vi "9-2.vi"() -> ()   [LabVIEW 2019, in "9.lvlib"]
uses:
  9.lvlib
panel:
  out "sum":i32
  out "number":i32[][](array[numeric])
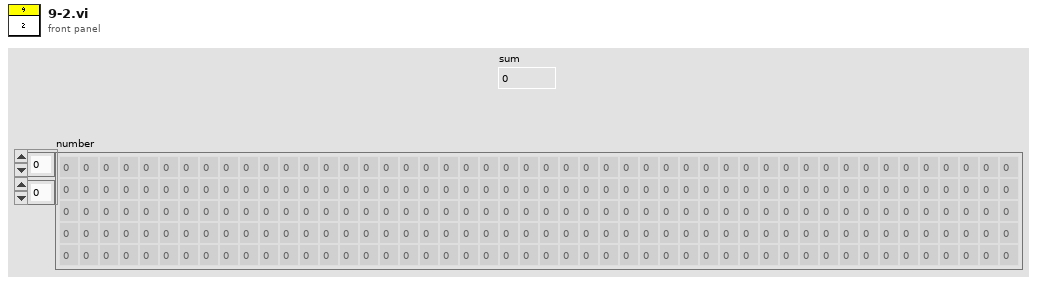
[diagram p1: front panel]
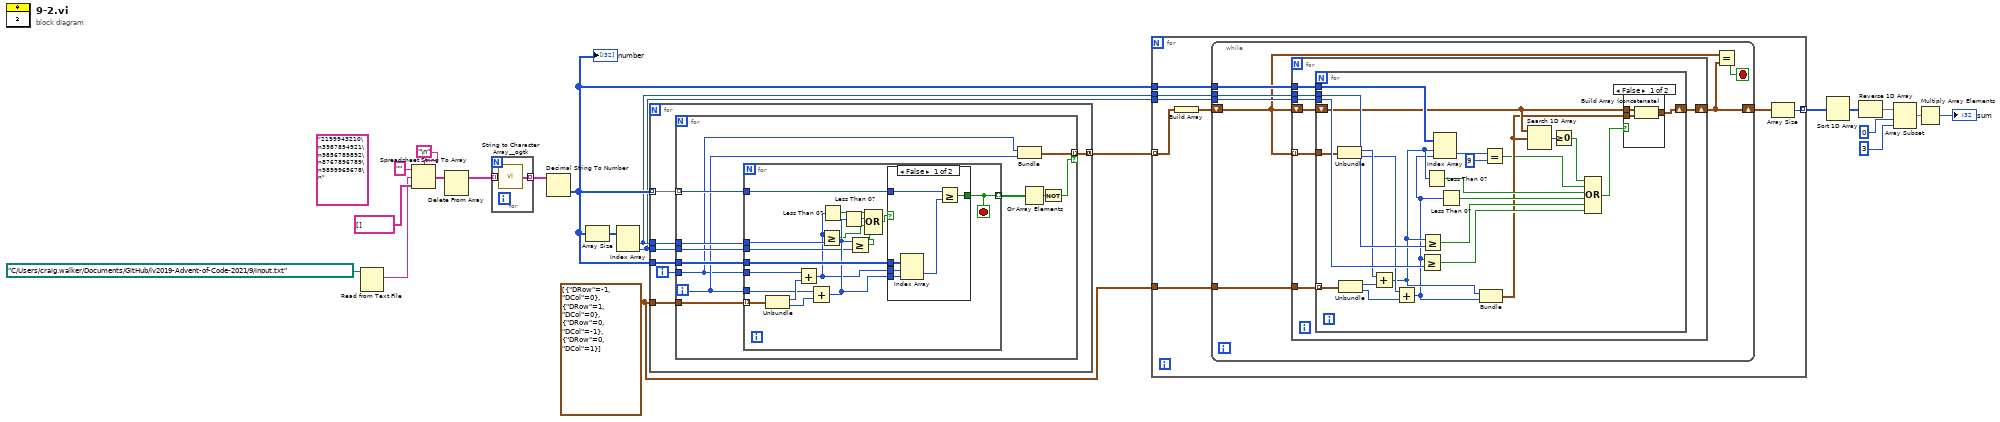
[diagram p0: block diagram]
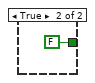
[diagram p3: hidden frame]
diagram:
  w9 = cluster{"DRow":i32, "DCol":i32}[] [{"DRow"=-1, "DCol"=0}, {"DRow"=1, "DCol"=0}, {"DRow"=0, "DCol"=-1}, {"DRow"=0, "DCol"=1}]
  (unwired) "2199943210\n3987894921\n9856789892\n8767896789\n9899965678\n"
  n1 = Read from Text File(file (use dialog)=path "C:/Users/craig.walker/Documents/GitHub/lv2019-Advent-of-Code-2021/9/input.txt") -> (text=w13:string)  [unwired: 3 in, 3 out]
  n2 = Spreadsheet String To Array(delimiter (Tab)="\n", format string="", spreadsheet string=w13, array type (2D Dbl)=string[] []) -> (array=w20:string[])
  n3 = Delete From Array(array=w20) -> (array with subset deleted=w14:string[])  [unwired: 2 in, 1 out]
  n4 = for {
    tunnel: w14 -> [w23] mode=indexing
    tunnel: [w22] -> w19 mode=indexing
    n5 = call <userlib>:"String to Character Array__ogtk.vi"("Input String"=w23) -> ("Character Array"=w22:string[])
  }
  n6 = Decimal String To Number(string=w19) -> (number=w12:i32[][])  [unwired: 2 in, 1 out]
  "number" <- w12
  n7 = Array Size(array=w12) -> (size(s)=w17:i32[])
  n8 = Index Array(array=w17) -> (element #1=w11:i32, element #2=w10:i32)  [unwired: 2 in]
  n9 = for {
    tunnel: w12 -> [w29] mode=indexing
    tunnel: w12 -> [w30]
    tunnel: w11 -> [w27]
    tunnel: w10 -> [w26]
    tunnel: w9 -> [w25]
    tunnel: [w24] -> w8 mode=concatenating
    i -> [w28]
    n10 = for {
      tunnel: w30 -> [w41]
      tunnel: w29 -> [w38] mode=indexing
      tunnel: w28 -> [w31]
      tunnel: w27 -> [w35]
      tunnel: w26 -> [w36]
      tunnel: w25 -> [w40]
      tunnel: [w32] -> w24 mode=indexing if=w34
      i -> [w33]
      n11 = for {
        tunnel: w41 -> [w50]
        tunnel: w31 -> [w56]
        tunnel: w33 -> [w54]
        tunnel: w40 -> [w58] mode=indexing
        tunnel: w38 -> [w48]
        tunnel: [w49] -> w39 mode=indexing
        tunnel: w36 -> [w46]
        tunnel: w35 -> [w45]
        stop <- w49 stop-if-true
        n12 = Unbundle(w58) -> ("DRow"=w57:i32, "DCol"=w55:i32)
        n13 = Add(x=w56, y=w57) -> (x+y=w44:i32)
        n14 = Add(x=w54, y=w55) -> (x+y=w47:i32)
        n15 = Greater Or Equal?(x=w44, y=w45) -> (x >= y?=w43:bool)
        n16 = Less Than 0?(x=w44) -> (x < 0?=w52:bool)
        n17 = Less Than 0?(x=w47) -> (x < 0?=w53:bool)
        n18 = Greater Or Equal?(x=w47, y=w46) -> (x >= y?=w42:bool)
        n19 = Compound Arithmetic op=OR(w52, w53, w43, w42) -> (w51:bool)
        n20 = case shown="False" w51 {
          tunnel: w48 -> [w64 _]
          tunnel: w50 -> [w63 _]
          tunnel: w44 -> [w62 _]
          tunnel: w47 -> [w61 _]
          tunnel: [w59 FALSE] -> w49
          frame False {
            n21 = Index Array(array=w63, index (row)=w62, index (col)=w61) -> (element=w60:i32)
            n22 = Greater Or Equal?(x=w64, y=w60) -> (x >= y?=w59:bool)
          }
          frame True {
          }
        }
      }
      n23 = Bundle(w31, w33) -> (w32:cluster{i32, i32})  [unwired: 1 in]
      n24 = Or Array Elements(Boolean array=w39) -> (logical OR=w37:bool)
      n25 = Not(x=w37) -> (.not. x?=w34:bool)
    }
  }
  n26 = for {
    tunnel: w8 -> [w69] mode=indexing
    tunnel: w12 -> [w73]
    tunnel: w11 -> [w72]
    tunnel: w10 -> [w71]
    tunnel: w9 -> [w70]
    tunnel: [w67] -> w7 mode=indexing
    n27 = Build Array(w69) -> (w68:cluster{i32, i32}[])
    n28 = while {
      tunnel: w73 -> [w80]
      tunnel: w72 -> [w79]
      tunnel: w71 -> [w78]
      tunnel: w70 -> [w77]
      shift-right: [w75] -> w66
      shift-left: w68 -> [w76]
      stop <- w74 stop-if-true
      n29 = for {
        tunnel: w80 -> [w87]
        tunnel: w79 -> [w86]
        tunnel: w78 -> [w85]
        tunnel: w77 -> [w84]
        tunnel: w76 -> [w81] mode=indexing
        shift-right: [w82] -> w75
        shift-left: w76 -> [w83]
        n30 = for {
          tunnel: w81 -> [w95]
          tunnel: w87 -> [w111]
          tunnel: w86 -> [w108]
          tunnel: w85 -> [w107]
          tunnel: w84 -> [w102] mode=indexing
          shift-right: [w97] -> w82
          shift-left: w83 -> [w96]
          n31 = Unbundle(w95) -> (w100:i32, w98:i32)
          n32 = Unbundle(w102) -> ("DRow"=w101:i32, "DCol"=w99:i32)
          n33 = Add(x=w100, y=w101) -> (x+y=w94:i32)
          n34 = Add(x=w98, y=w99) -> (x+y=w93:i32)
          n35 = Greater Or Equal?(x=w93, y=w107) -> (x >= y?=w103:bool)
          n36 = Greater Or Equal?(x=w94, y=w108) -> (x >= y?=w105:bool)
          n37 = Less Than 0?(x=w94) -> (x < 0?=w104:bool)
          n38 = Index Array(array=w111, index (row)=w94, index (col)=w93) -> (element=w110:i32)
          n39 = Less Than 0?(x=w93) -> (x < 0?=w106:bool)
          n40 = Bundle(w94, w93) -> (w92:cluster{i32, i32})  [unwired: 1 in]
          n41 = Equal?(x=w110, y=9) -> (x = y?=w89:bool)
          n42 = Search 1D Array(1D array=w96, element=w92) -> (index of element=w91:i32)  [unwired: 1 in]
          n43 = Greater Or Equal To 0?(x=w91) -> (x >= 0?=w90:bool)
          n44 = Compound Arithmetic op=OR(w90, w89, w104, w106, w105, w103) -> (w88:bool)
          n45 = case shown="False" w88 {
            tunnel: w92 -> [w114 _]
            tunnel: [w113 w115] -> w97
            tunnel: w96 -> [w112 w115]
            frame False {
              n46 = Build Array (concatenate)(w112, w114) -> (w113:cluster{i32, i32}[])
            }
            frame True {
            }
          }
        }
      }
      n47 = Equal?(x=w76, y=w75) -> (x = y?=w74:bool)
    }
    n48 = Array Size(array=w66) -> (size(s)=w67:i32)
  }
  n49 = Sort 1D Array(array=w7) -> (sorted array=w6:i32[])
  n50 = Reverse 1D Array(array=w6) -> (reversed array=w5:i32[])
  n51 = Array Subset(array=w5, index=0, length=3) -> (w2:i32[])
  n52 = Multiply Array Elements(1:w2) -> (0:→"sum":i32)
